vi "添加单引号.vi"(8 "error in (no error)":errorcluster caption="错误输入（无错误）", 11 "string":string caption="字符串") -> (0 "error out":errorcluster caption="错误输出", 3 "with quotes":string caption="包括引号")   [LabVIEW 2012]
doc: "Adds quote marks (\") around a string that contains spaces."
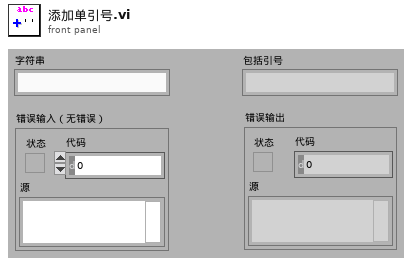
[diagram p1: front panel]
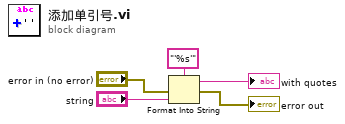
[diagram p0: block diagram]
diagram:
  n1 = Format Into String(format string="'%s'", error in="error in (no error)", "string") -> (resulting string=→"with quotes":string, error out=→"error out":errorcluster)  [unwired: 1 in]
